vi "Examen.vi"() -> ()   [LabVIEW 2020]
uses:
  <vilib>/numeric/Random Number (Range) U64.vi
  <vilib>/numeric/sub_Random U32.vi
panel:
  out "Numeros que han superado el maximo":dbl
  out "Datos filtrados":dbl[](array[numeric])
  out "Datos":dbl[](array[numeric])
  out "Waveform Graph":dynamicdata(graph)
  in  "Finalizar y guardar datos":bool
  in  "Máximo 2":dbl
  in  "Mínimo":dbl
  out "Rango\n 2":bool
  out "Histeresis 2":bool
  out "Señal analógica":dbl
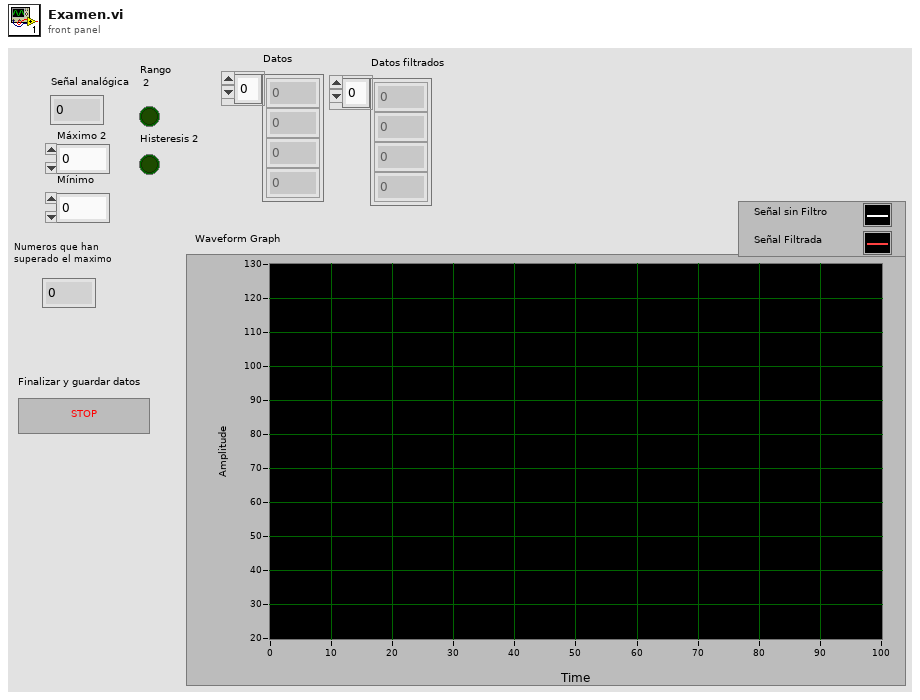
[diagram p1: front panel]
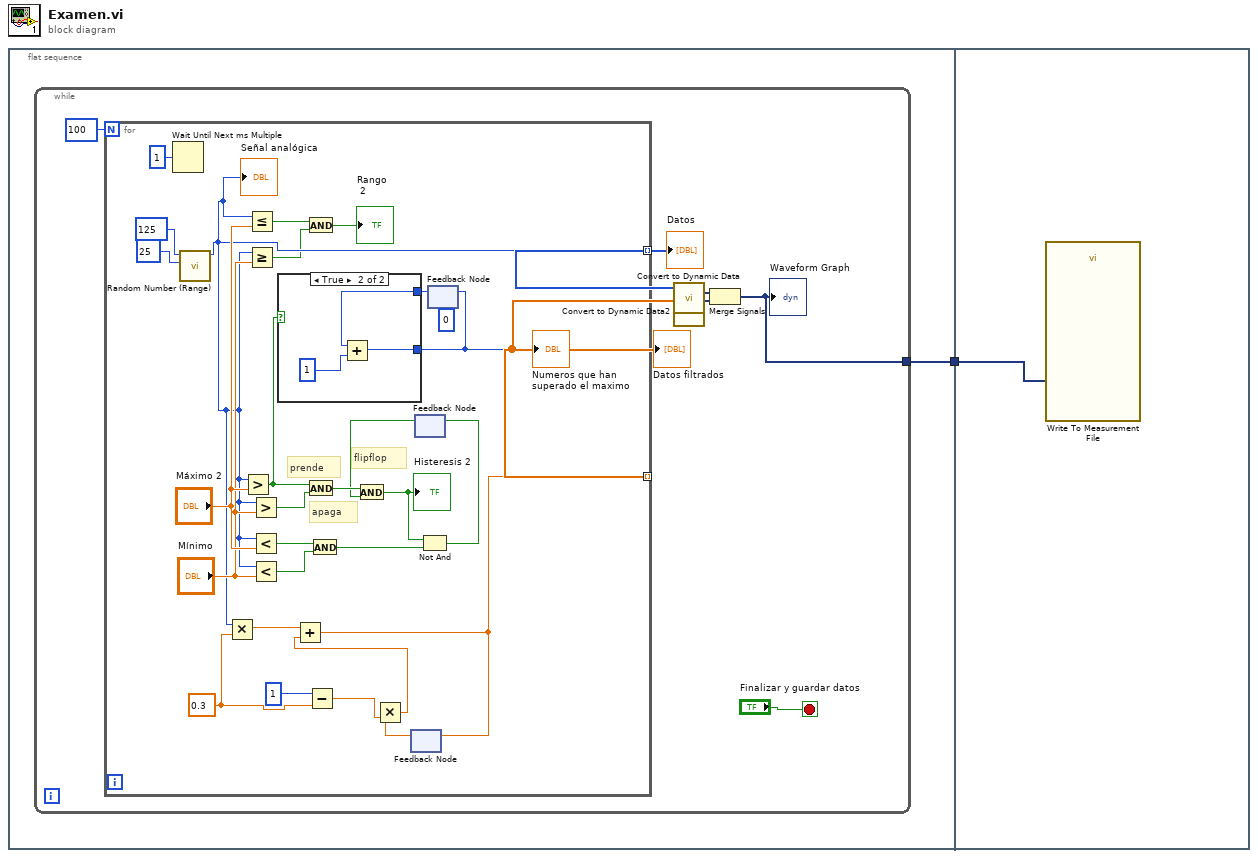
[diagram p0: block diagram]
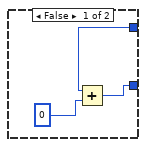
[diagram p2: hidden frame]
diagram:
  n1 = flat-sequence {
    tunnel: [w2] -> w1
    tunnel: w1 -> [w44]
    frame #0 {
      n2 = while {
        tunnel: [w3] -> w2
        stop <- "Finalizar y guardar datos" stop-if-true
        n3 = for {
          N: 100 -> [_]
          tunnel: [w16] -> w8 mode=indexing
          tunnel: [w15] -> w6 mode=indexing
          w20 = 0.3
          # "flipflop"
          # "apaga"
          # "prende"
          n4 = Wait Until Next ms Multiple(millisecond multiple=u32 1) -> ()  [unwired: 1 out]
          n5 = call-poly <vilib>:"Random Number (Range).vi"("lower bound (0)"=u64 25, "upper bound (100)"=u64 125) -> ("number"=w16:u64)  [unwired: 9 in]
          "Señal analógica" <- w16
          n6 = Multiply(x=w16, y=w20) -> (x*y=w22:dbl)
          n7 = Greater?(x=w16, y="Máximo 2") -> (0:w13:bool)
          n8 = Less Or Equal?(x=w16, y="Máximo 2") -> (x <= y?=w34:bool)
          n9 = Greater Or Equal?(x=w16, y="Mínimo") -> (x >= y?=w14:bool)
          n10 = Greater?(x=w16, y="Mínimo") -> (0:w25:bool)
          n11 = Less?(x=w16, y="Máximo 2") -> (x < y?=w31:bool)
          n12 = Less?(x=w16, y="Mínimo") -> (x < y?=w30:bool)
          n13 = And(x=w34, y=w14) -> (x .and. y?=→"Rango\n 2":bool)
          n14 = And(x=w13, y=w25) -> (x .and. y?=w29:bool)
          n15 = Subtract(x=1, y=w20) -> (x-y=w18:dbl)
          n16 = And(x=w31, y=w30) -> (x .and. y?=w28:bool)
          n17 = feedback #1() -> (w17:dbl)  [unwired: 1 in]
          n18 = Multiply(x=w17, y=w18) -> (x*y=w19:dbl)
          n19 = Add(x=w22, y=w19) -> (x+y=w15:dbl)
          n20 = feedback-in #1(w15) -> ()
          n21 = feedback #2() -> (w23:bool)  [unwired: 1 in]
          n22 = And(x=w29, y=w23) -> (x .and. y?=w27:bool)
          "Histeresis 2" <- w27
          n23 = Not And(1:w28, 2:w27) -> (0:w24:bool)
          n24 = feedback-in #2(w24) -> ()
          n25 = feedback #3(0) -> (w12:i32)
          n26 = case shown="True" w13 {
            tunnel: w12 -> [w38 w42]
            tunnel: [w39 w41] -> w10
            frame False {
              n27 = Add(x=w38, y=0) -> (x+y=w39:i32)
            }
            frame True {
              n28 = Add(x=w42, y=1) -> (x+y=w41:i32)
            }
          }
          "Numeros que han superado el maximo" <- w10
          n29 = feedback-in #3(w10) -> ()
        }
        "Datos" <- w8
        "Datos filtrados" <- w6
        n30 = call "Convert to Dynamic Data"("Array"=w8) -> ("Dynamic Data Type"=w7:dynamicdata)  [unwired: 3 in]
        n31 = call "Convert to Dynamic Data2"("Array"=w6) -> ("Dynamic Data Type"=w5:dynamicdata)  [unwired: 3 in]
        n32 = Merge Signals(w7, w5) -> (w3:dynamicdata)
        "Waveform Graph" <- w3
      }
    }
    frame #1 {
      n33 = call "Write To Measurement File"("Signals"=w44) -> ()  [unwired: 16 in, 3 out]
    }
  }
